vi "CFTS-Change Password Dialog.vi"(2 "Parent VI":refnum<vi>) -> (8 "hash":string)   [LabVIEW 2020]
uses:
  <vilib>/security/Message Digest/API/Instances/Byte Array/SHA-256 Byte Array Checksum.vi
  <vilib>/security/Message Digest/API/NI_Message Digest API.lvlib
panel:
  in  "Reenter":string
  in  "Enter password":string
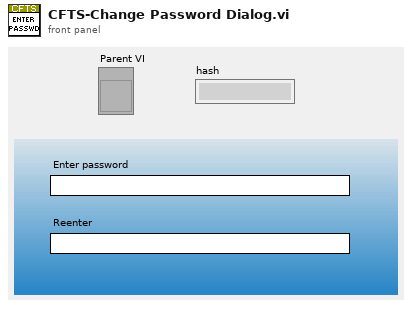
[diagram p1: front panel]
types:
  T1 = enum8{"Enabled", "Disabled", "Disabled and Grayed Out"}
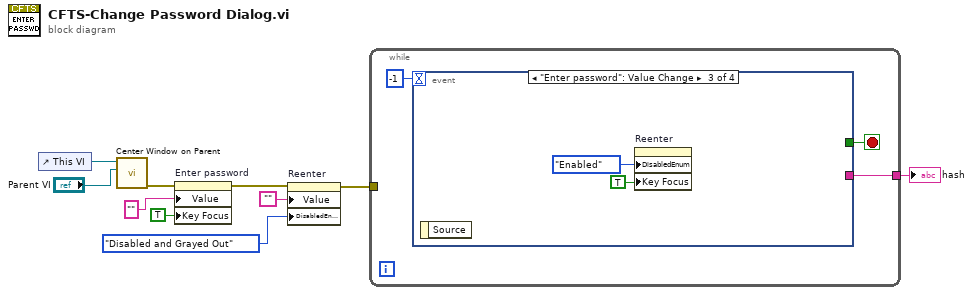
[diagram p0: block diagram]
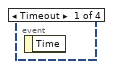
[diagram p2: hidden frame]
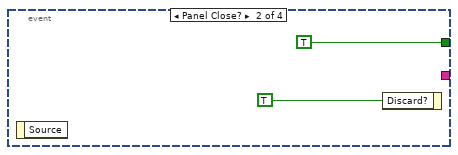
[diagram p3: hidden frame]
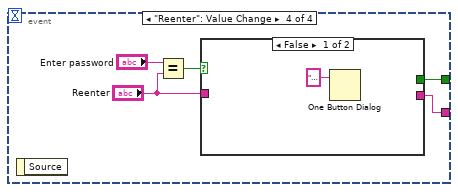
[diagram p4: hidden frame]
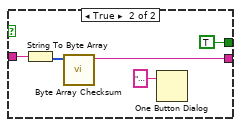
[diagram p5: hidden frame]
diagram:
  n1 = control-ref of="This VI"() -> (w9:refnum<vi>)
  n2 = call "Center Window on Parent.vi"("Parent VI"="Parent VI", "VI in"=w9) -> ("error out"=w7:errorcluster)  [unwired: 8 in, 1 out]
  n3 = property on="Enter password" class="Str"(error in=w7, "Value"="" ("Enter password"), "Key Focus"=TRUE) -> (error out=w4:errorcluster)  [unwired: 1 in, 1 out]
  n4 = property on="Reenter" class="Str"(error in=w4, "Value"="", "DisabledEnum"=T1."Disabled and Grayed Out" ("Disabled")) -> (error out=w3:errorcluster)  [unwired: 1 in, 1 out]
  n5 = while {
    tunnel: [w11] -> w10
    tunnel: w3 -> [_]
    stop <- w12 stop-if-true
    n6 = event shown="[2] \"Enter password\": Value Change" {
      selector: _ -> [_ _ _ _]
      dyn-events: _ -> [_ _ _ _]
      timeout: -1 -> [_ _ _ _]
      tunnel: [_ TRUE _ w18] -> w12
      tunnel: [_ _ _ w19] -> w11
      event Timeout {
        n7 = event-data() -> ()  [unwired: 1 in, 1 out]
      }
      event Panel Close? {
        n8 = event-data() -> ()  [unwired: 1 in, 1 out]
        n9 = event-data("Discard?"=TRUE) -> ()  [unwired: 1 in, 1 out]
      }
      event "Enter password": Value Change {
        n10 = event-data() -> ()  [unwired: 1 in, 1 out]
        n11 = property on="Reenter" class="Str"("DisabledEnum"=T1."Enabled" ("Disabled"), "Key Focus"=TRUE) -> ()  [unwired: 2 in, 2 out]
      }
      event "Reenter": Value Change {
        n12 = event-data() -> ()  [unwired: 1 in, 1 out]
        n13 = Equal?(x="Enter password", y="Reenter") -> (x = y?=w21:bool)
        n14 = case shown="False" w21 {
          tunnel: "Reenter" -> [_ w27]
          tunnel: [_ w26] -> w19
          tunnel: [_ TRUE] -> w18
          frame False {
            n15 = One Button Dialog(message="Passwords do not match!") -> ()  [unwired: 1 in, 1 out]
          }
          frame True {
            n16 = String To Byte Array(string=w27) -> (unsigned byte array=w28:u8[])
            n17 = call-poly <vilib>:"Byte Array Checksum.vi"("buffer"=w28) -> ("digest"=w26:string)  [unwired: 10 in]
            n18 = One Button Dialog(message="Password changed") -> ()  [unwired: 1 in, 1 out]
          }
        }
      }
    }
  }
  "hash" <- w10
